vi "Read Width (us).vi"(8 "error in (no error)":errorcluster, 11 "Pulse Train in":refnum<class "Pulse Train.lvclass">) -> (0 "error out":errorcluster, 2 "Width (us)":string, 3 "Pulse Train out":refnum<class "Pulse Train.lvclass">)   [LabVIEW 2020, in "Pulse Train.lvclass"]
uses:
  Pulse Train.lvclass
  Pulse Train.lvclass/Pulse Train.ctl
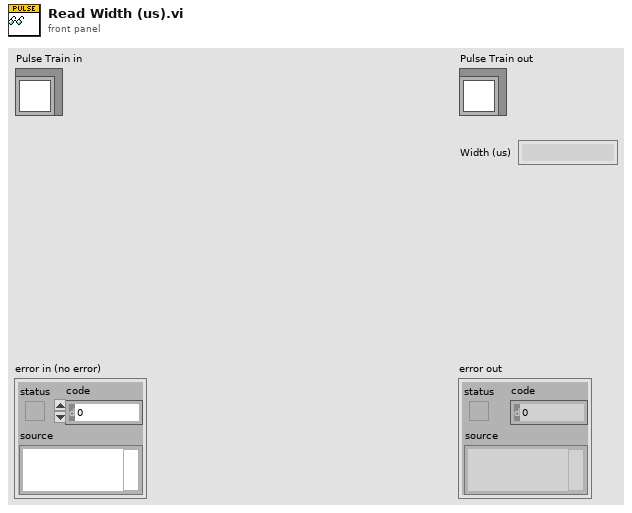
[diagram p1: front panel]
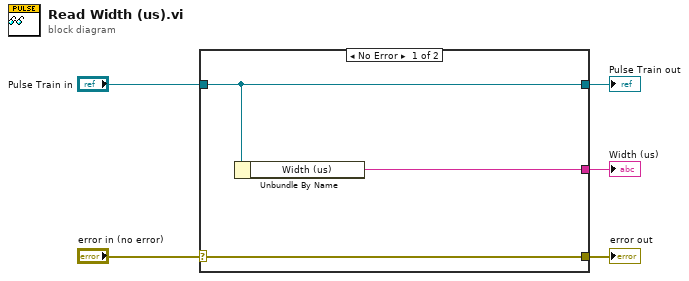
[diagram p0: block diagram]
diagram:
  n1 = case shown="No Error" "error in (no error)" {
    selector: "error in (no error)" -> [w8 w9]
    tunnel: [w8 w9] -> w4
    tunnel: [w7 w10] -> w2
    tunnel: "Pulse Train in" -> [w7 w10]
    tunnel: [w6 _] -> w1
    frame No Error {
      n2 = Unbundle By Name(w7) -> ("Width (us)"=w6:string)
    }
    frame Error {
    }
  }
  "error out" <- w4
  "Pulse Train out" <- w2
  "Width (us)" <- w1
